vi "Receive User Menu Selection Event.vi"(8 "error in (no error)":errorcluster, 10 "MenuSelectionMsg":refnum<class "MenuSelectionMsg.lvclass">, 11 "ActorAutoRegistrationView In":refnum<class "EventHandlingActor.lvclass">) -> (0 "error out":errorcluster, 3 "ActorAutoRegistrationView Out":refnum<class "EventHandlingActor.lvclass">)   [LabVIEW 2018, in "TestViewables.lvlib" / "EventHandlingActor.lvclass"]
doc: "<License>\nCopyright © 2017 Composed Systems, LLC | All rights reserved\nwww.composed.io\n\nAuthor: Ethan Stern <ethan.stern@composed.io>\n\nThis software is provided \"AS IS\" WITHOUT WARRANTIES, either express or implied, AND IS FOR EDUCATIONAL PURPOSES ONLY.\n</License>"
uses:
  EventHandlingActor.lvclass
  Source/DialogBox/OneButtonDialogBox/OneButtonDialogBox.lvclass
  modules/mva-viewable/Source/ActorEvents/IEventAggregator Messages/MenuSelectionMsg/MenuSelectionMsg.lvclass
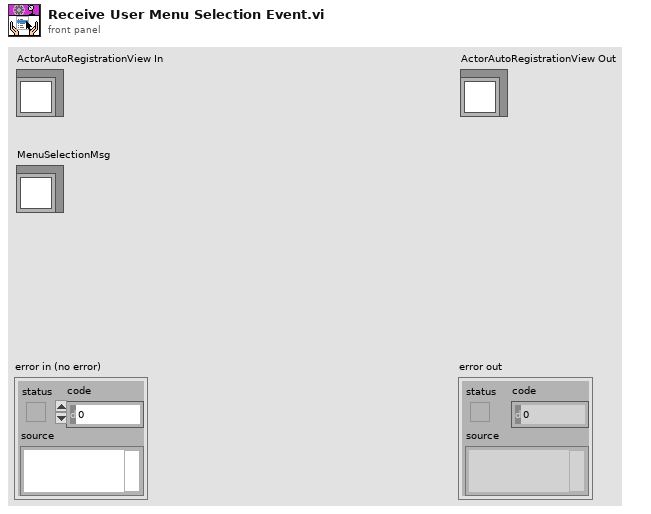
[diagram p1: front panel]
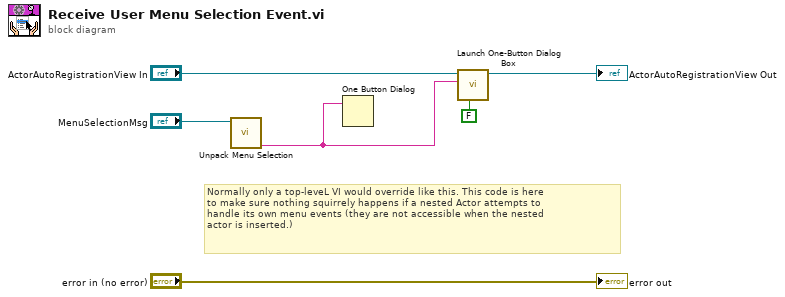
[diagram p0: block diagram]
diagram:
  # "Normally only a top-leveL VI would override like this. This code is here\nto make sure nothing squirrely happens if a nested Actor attempts to\nhandle its own menu events (they are not accessible when the nested\nactor is inserted.)"
  n1 = call "Unpack Menu Selection.vi"("MenuSelectionMsg"="MenuSelectionMsg") -> ("Item Tag"=w1:string)  [unwired: 5 in, 5 out]
  n2 = One Button Dialog(message=w1) -> ()  [unwired: 1 in, 1 out]
  n3 = call "Launch One-Button Dialog Box.vi"("Modal? (T)"=FALSE, "Message Text"=w1, "Dialog Launcher"="ActorAutoRegistrationView In") -> ("Dialog Launcher Out"=→"ActorAutoRegistrationView Out":refnum<class "EventHandlingActor.lvclass">)  [unwired: 7 in, 1 out]
  "error out" <- "error in (no error)"
